vi "derivative.vi"(1 "Time Constant":dbl, 2 "dt_ms":dbl, 3 "IC":bool, 4 "Input":dbl) -> (0 "Output":dbl)   [LabVIEW 2025]
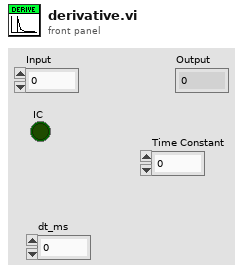
[diagram p1: front panel]
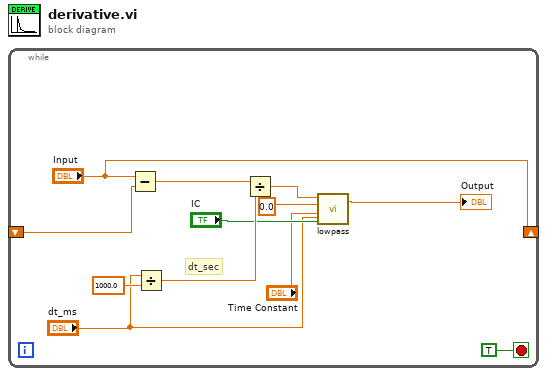
[diagram p0: block diagram]
diagram:
  n1 = while {
    shift-right: ["Input"] -> _
    shift-left: _ -> [w11]
    stop <- TRUE stop-if-true
    # "dt_sec"
    n2 = Subtract(x="Input", y=w11) -> (x-y=w7:dbl)
    n3 = Divide(x="dt_ms", y=1000.0) -> (x/y=w10:dbl)
    n4 = Divide(x=w7, y=w10) -> (x/y=w9:dbl)
    n5 = call "lowpass.vi"("MS"="dt_ms", "Boolean"="IC", "TC"="Time Constant", "IC Value"=0.0, "In"=w9) -> ("Out"=→"Output":dbl)
  }
